vi "Switch_Manager_SoftFP.vi"(0 "reference in":refnum<class "Switch_Manager.lvclass">, 2 "Floating":bool, 5 "error in (no error)":errorcluster) -> (14 "reference out":refnum<class "Switch_Manager.lvclass">, 19 "error out":errorcluster)   [LabVIEW 2022 SP3, in "Switch_Manager.lvlib" / "Switch_Manager.lvclass"]
uses:
  Switch_Manager.lvclass
  <vilib>/picture/picture.llb/imagedata.ctl
  Components/ViPER.lvlibp/ViPER.lvclass
  C:/Projects/Medulla/ViPER/Examples/Flux_Capacitor_Tester/Components/ViPER.lvlibp/ViPER.lvclass
panel:
  in  "Disconnect":bool
  in  "Connect":bool
  in  "Tree":string(tree)
  in  "Disconnect_All":bool
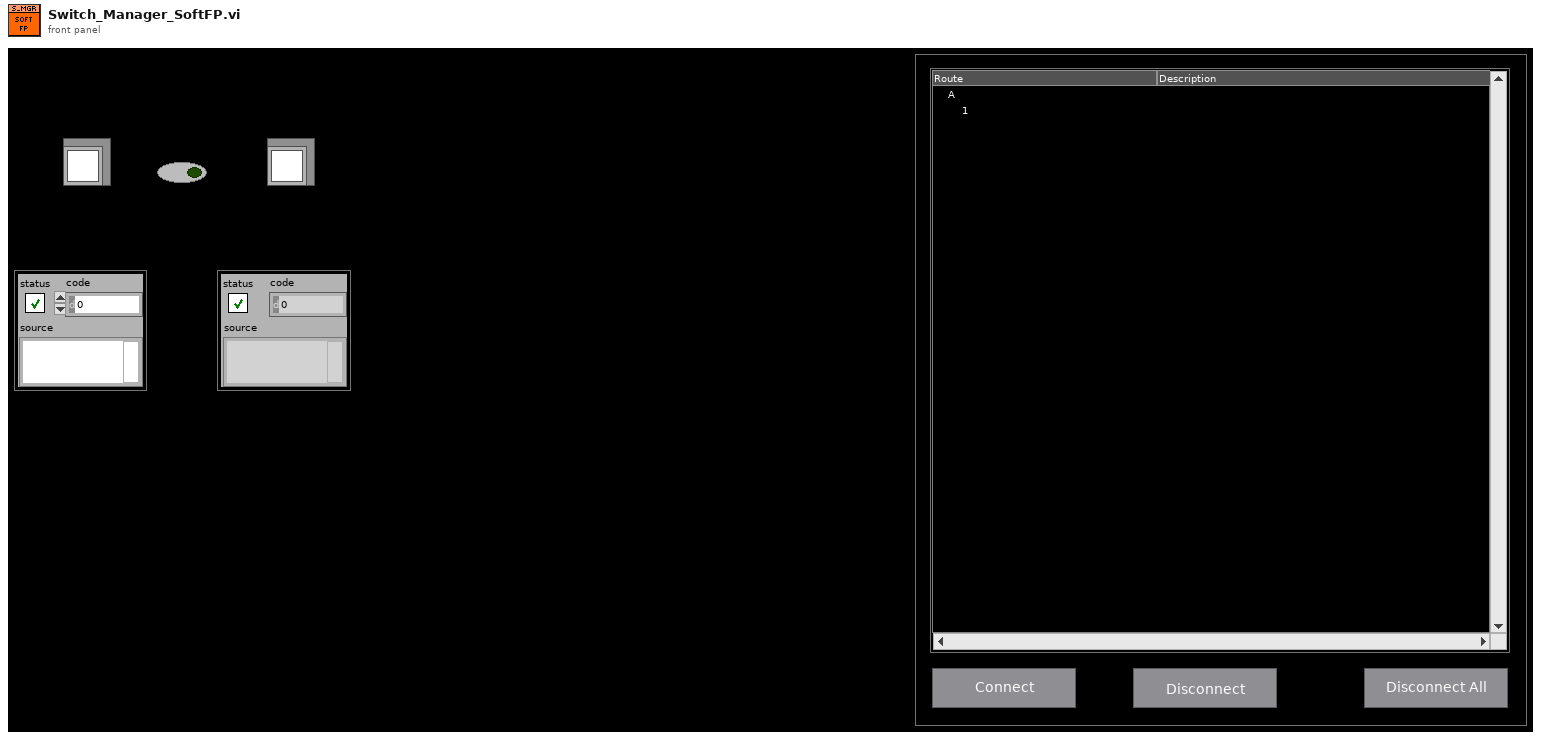
[diagram p1: front panel]
types:
  T1 = enum32{"Invalid", "Standard", "Closed", "Hidden", "Minimized", "Maximized"}
  T2 = typedef "Switch_Manager.lvlib/Switch_Manager.lvclass/ObjectAttributes.ctl" = cluster{"Config":T3, "State":bool[], "Switches":refnum<class "SwitchBase.lvclass">[], "SwitchName":string[], "SwitchMap":T4[], "UpdateEvent":refnum<user-event>, "ParentEvent":refnum<user-event>, "Tree":bool[]}
  T3 = typedef "Switch_Manager.lvlib/Switch_Manager.lvclass/Config.ctl" = cluster{"default":string}
  T4 = typedef "Switch_Manager.lvlib/Switch_Manager.lvclass/SwitchMap.ctl" = cluster{"Name":string, "Description":string, "Group":string, "IsGroup":bool, "Switches":string[]}
  T5 = typedef "imagedata.ctl" = cluster{"image type":i32, "image depth":i32, "image":u8[], "mask":u8[], "colors":u32[], "Rectangle":cluster{"left":i16, "top":i16, "right":i16, "bottom":i16}}
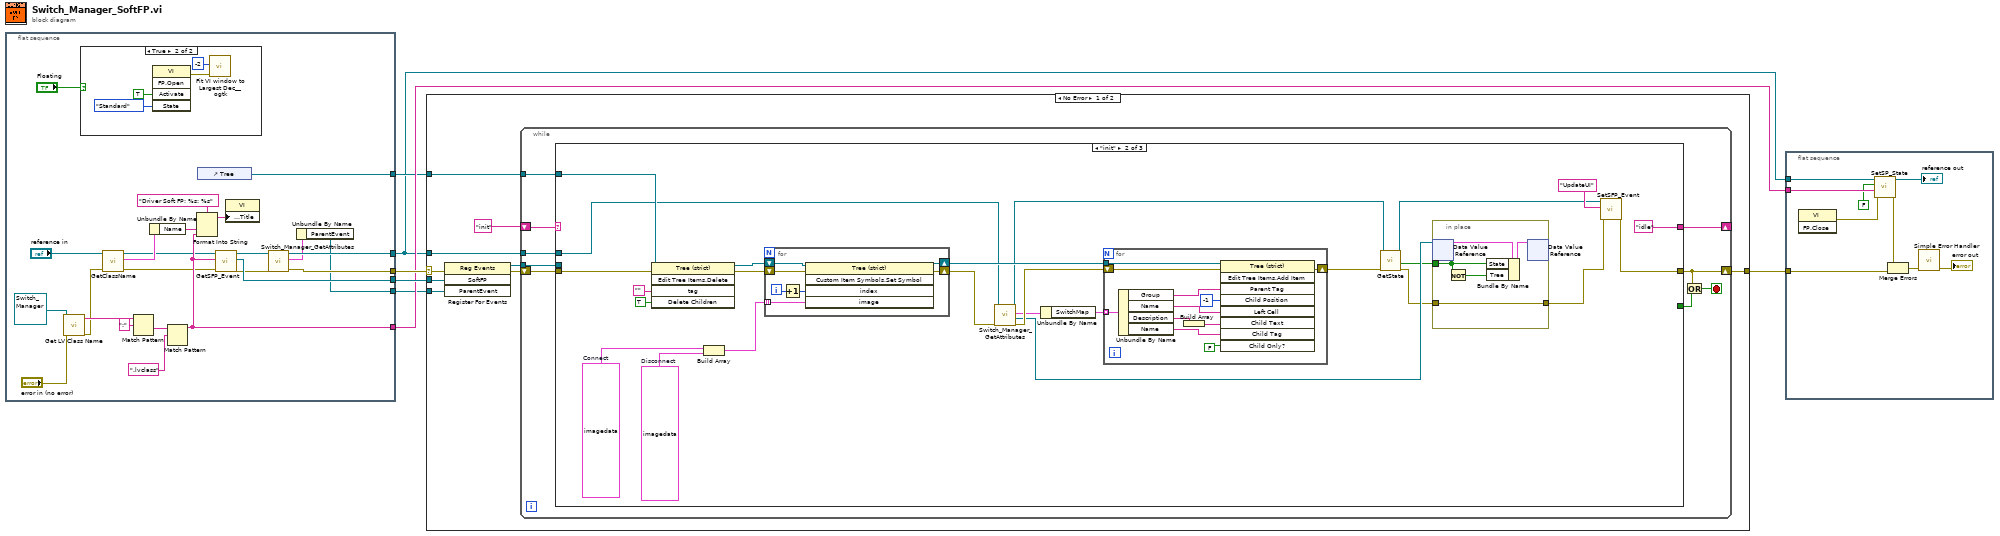
[diagram p0: block diagram]
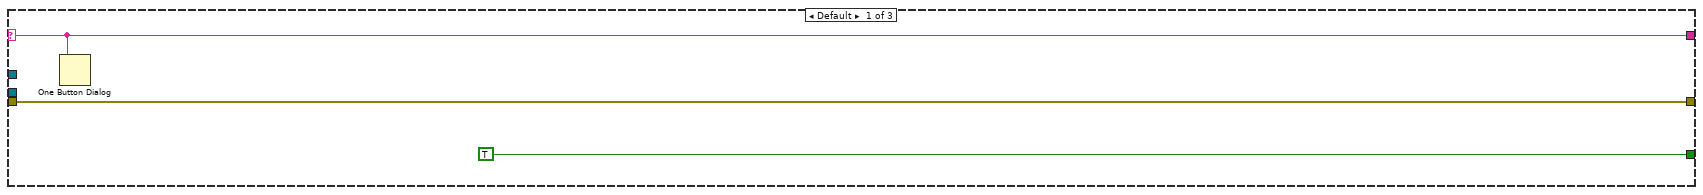
[diagram p3: hidden frame]
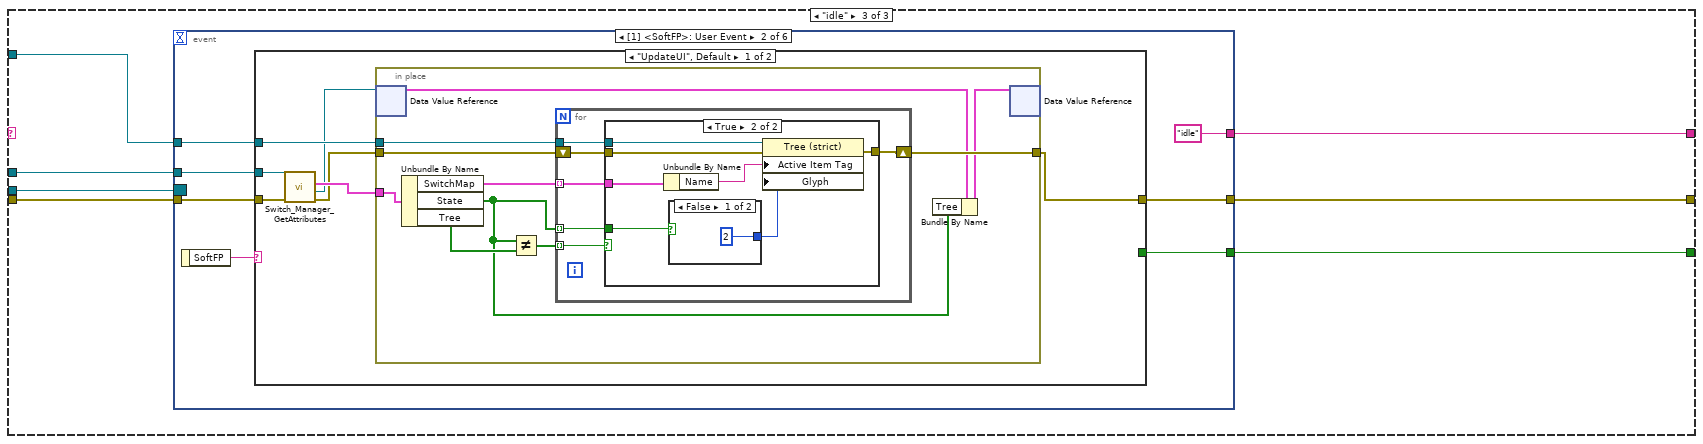
[diagram p4: hidden frame]
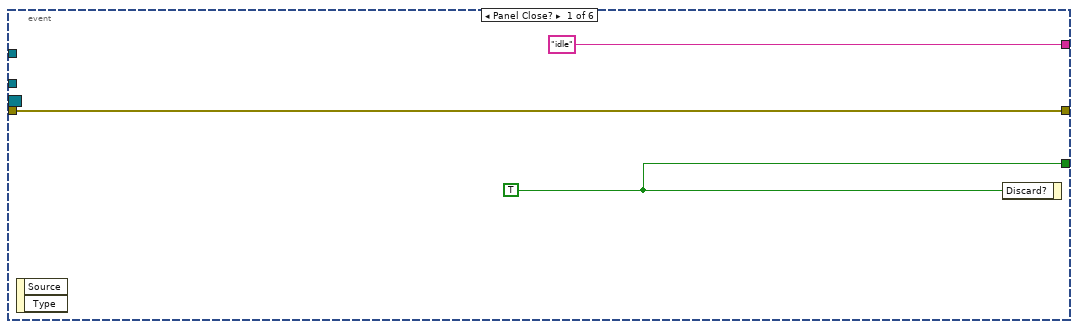
[diagram p5: hidden frame]
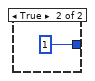
[diagram p7: hidden frame]
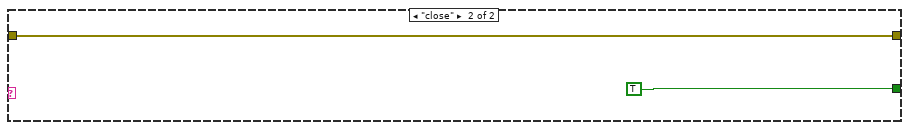
[diagram p8: hidden frame]
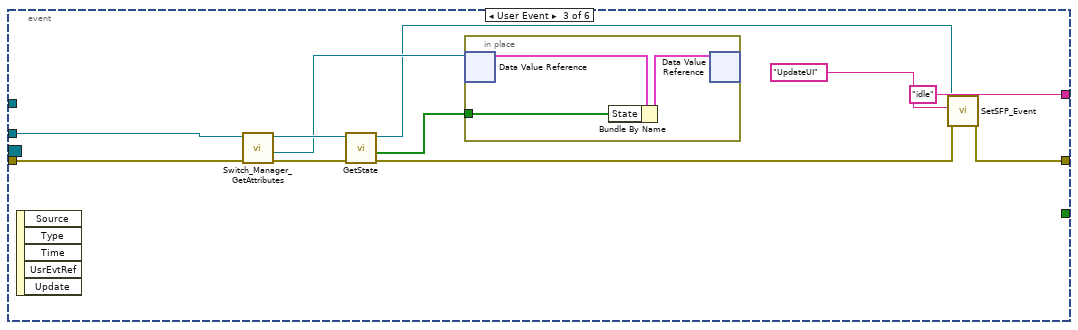
[diagram p9: hidden frame]
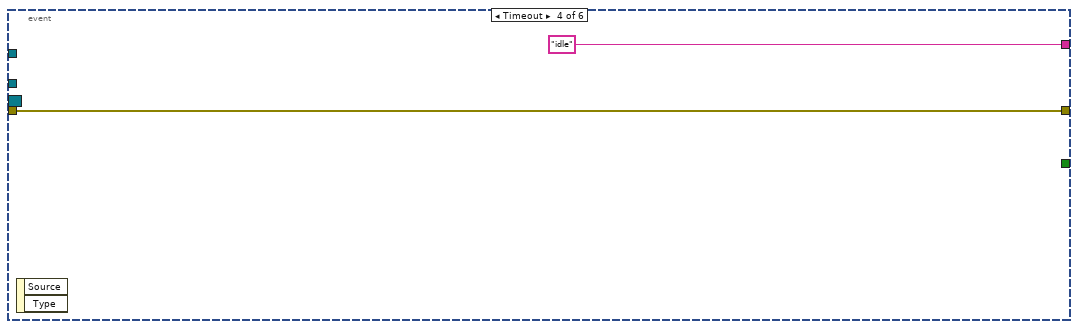
[diagram p10: hidden frame]
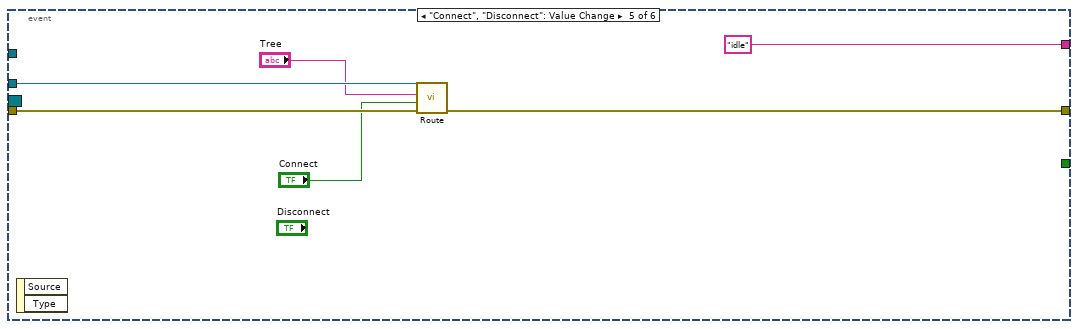
[diagram p11: hidden frame]
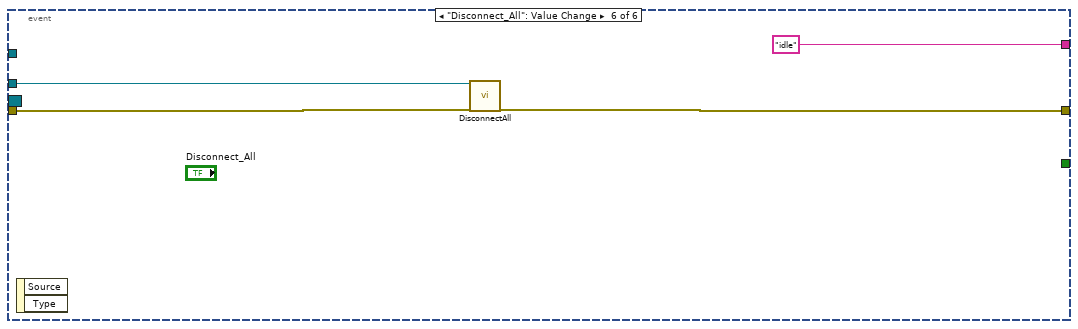
[diagram p12: hidden frame]
diagram:
  n1 = flat-sequence {
    tunnel: [w12] -> w7
    tunnel: [w10] -> w2
    tunnel: [w31] -> w5
    tunnel: [w21] -> w4
    tunnel: [w14] -> w3
    tunnel: [w8] -> w1
    frame #0 {
      n2 = call <vilib>:"Get LV Class Name.vi"("error in (no error)"="error in (no error)", "object"=refnum<class "Switch_Manager.lvclass"> refnum ("reference")) -> ("error out"=w20:errorcluster, "class name"=w26:string)  [unwired: 8 in]
      n3 = case shown="True" "Floating" {
        frame False {
        }
        frame True {
          n4 = invoke class="VI" method="FP.Open"("Activate"=TRUE ("Activate?"), "State"=T1."Standard") -> (error out=w32:errorcluster)  [unwired: 3 in, 4 out]
          n5 = call <userlib>:"Fit VI window to Largest Dec__ogtk.vi"("error in (no error)"=w32, "border spacing (2 px)"=-2) -> ()  [unwired: 4 in, 2 out]
        }
      }
      n6 = call "GetClassName.vi"("error in (no error)"=w20, "reference in"="reference in") -> ("error out"=w19:errorcluster, "Details"=w18:cluster{"Name":string, "Class":string}, "reference out"=w16:refnum<class "Switch_Manager.lvclass">)  [unwired: 7 in]
      n7 = Match Pattern(string=w26, regular expression=":") -> (after substring=w24:string)  [unwired: 1 in, 3 out]
      n8 = Unbundle By Name(w18) -> ("Name"=w28:string)
      n9 = Match Pattern(string=w24, regular expression=".lvclass") -> (before substring=w21:string)  [unwired: 1 in, 3 out]
      n10 = Format Into String(format string="Driver Soft FP: %s: %s", w28, w21) -> (resulting string=w30:string)  [unwired: 2 in, 1 out]
      n11 = control-ref of="Tree"() -> (w14:refnum<vi>)
      n12 = call-dynamic "GetSFP_Event.vi"("error in (no error)"=w19, "Ancestor"=w21, "reference in"=w16) -> ("error out"=w13:errorcluster, "SoftFP"=w31:refnum<user-event>, "reference out"=w11:refnum<class "Switch_Manager.lvclass">)  [unwired: 6 in]
      n13 = property class="VI"("Front Panel.Title"=w30) -> ()  [unwired: 2 in, 2 out]
      n14 = call "Switch_Manager_GetAttributes.vi"("error in (no error)"=w13, "reference in"=w11) -> ("error out"=w12:errorcluster, "Data"=w9:T2, "reference out"=w10:refnum<class "Switch_Manager.lvclass">)  [unwired: 6 in, 1 out]
      n15 = Unbundle By Name(w9) -> ("ParentEvent"=w8:refnum<user-event>)
    }
  }
  n16 = case shown="No Error" w7 {
    selector: w7 -> [w42 w183]
    tunnel: [w38 w183] -> w6
    tunnel: w2 -> [w39 _]
    tunnel: w5 -> [w44 _]
    tunnel: w3 -> [w37 _]
    tunnel: w1 -> [w36 _]
    frame No Error {
      n17 = register-events(error in=w42, w44, w36) -> (reference out=w43:refnum<event-registration>, error out=w41:errorcluster)  [unwired: 1 in]
      n18 = while {
        shift-right: [w50] -> w38
        shift-left: w41 -> [w53]
        tunnel: w43 -> [w52]
        tunnel: w39 -> [w51]
        shift-right: [w46] -> _
        shift-left: "init" -> [w47]
        tunnel: w37 -> [w45]
        stop <- w49 stop-if-true
        n19 = case shown="\"init\"" w47 {
          selector: w47 -> [w54 _ _]
          tunnel: w53 -> [w55 w71 w111]
          tunnel: w52 -> [_ _ w110]
          tunnel: w51 -> [_ w66 w109]
          tunnel: [w55 w80 w108] -> w50
          tunnel: [TRUE ("Discard?") _ w107] -> w48
          tunnel: [w54 "idle" w106] -> w46
          tunnel: w45 -> [_ w70 w105]
          frame Default {
            n20 = One Button Dialog(message=w54) -> ()  [unwired: 1 in, 1 out]
          }
          frame "init" {
            w72 = T5 {"image type"=0, "image depth"=32, "image"=[255, 0, 0, 0, 255, 0, 0, 0, 255, 0, 0, 0, 255, 0, 0, 0, 255, 0, 0, 0, 255, 0, 0, 0, 255, 0, 0, 0, 255, 0, 0, 0, 255, 0, 0, 0, 255, 0, 0, 0, 255, 0, 0, 0, 255, 0, 0, 0, 255, 0, 0, 0, 255, 0, 0, 0, 255, 0, 0, 0, 255, 0, 0, 0, 255, 0, 0, 0, 255, 0, 0, 0, 255, 0, 0, 0, 255, 0, 0, 0, 255, 136, 118, 121, 255, 113, 64, 72, 255, 122, 43, 52, 255, 138, 48, 56, 255, 136, 46, 54, 255, 120, 40, 49, 255, 113, 64, 72, 255, 0, 0, 0, 255, 0, 0, 0, 255, 0, 0, 0, 255, 0, 0, 0, 255, 0, 0, 0, 255, 0, 0, 0, 255, 0, 0, 0, 255, 0, 0, 0, 255, 119, 79, 86, 255, 137, 51, 59, 255, 189, 85, 89, 255, 201, 100, 103, 255, 201, 102, 105, 255, 198, 94, 97, 255, 194, 81, 84, 255, 180, 64, 69, 255, 130, 39, 48, 255, 121, 84, 90, 255, 0, 0, 0, 255, 0, 0, 0, 255, 0, 0, 0, 255, 0, 0, 0, 255, 0, 0, 0, 255, 119, 79, 86, 255, 161, 64, 71, 255, 202, 103, 106, 255, 209, 123, 126, 255, 211, 129, 132, 255, 208, 122, 125, 255, 203, 105, 109, 255, 196, 87, 90, 255, 192, 74, 78, 255, 189, 68, 72, 255, 150, 47, 54, 255, 121, 86, 92, 255, 0, 0, 0, 255, 0, 0, 0, 255, 0, 0, 0, 255, 136, 118, 121, 255, 137, 51, 59, 255, 202, 103, 106, 255, 211, 129, 132, 255, 214, 140, 142, 255, 212, 133, 136, 255, 205, 113, 116, 255, 196, 88, 92, 255, 190, 68, 72, 255, 188, 63, 67, 255, 189, 68, 72, 255, 190, 69, 73, 255, 129, 40, 49, 255, 0, 0, 0, 255, 0, 0, 0, 255, 0, 0, 0, 255, 113, 64, 72, 255, 188, 84, 88, 255, 207, 120, 122, 255, 213, 135, 138, 255, 211, 131, 133, 255, 205, 112, 115, 255, 195, 85, 88, 255, 186, 59, 63, 255, 181, 44, 48, 255, 181, 45, 49, 255, 187, 61, 65, 255, 191, 73, 77, 255, 177, 62, 67, 255, 114, 68, 76, 255, 0, 0, 0, 255, 0, 0, 0, 255, 122, 42, 51, 255, 199, 94, 98, 255, 207, 118, 121, 255, 207, 119, 122, 255, 201, 102, 105, 255, 193, 78, 82, 255, 185, 54, 58, 255, 178, 36, 41, 255, 176, 28, 33, 255, 178, 34, 39, 255, 185, 55, 59, 255, 192, 74, 78, 255, 191, 71, 75, 255, 117, 40, 50, 255, 0, 0, 0, 255, 0, 0, 0, 255, 136, 44, 53, 255, 197, 89, 92, 255, 201, 100, 103, 255, 197, 88, 92, 255, 189, 67, 71, 255, 182, 47, 52, 255, 177, 33, 38, 255, 174, 25, 30, 255, 174, 23, 28, 255, 177, 32, 37, 255, 185, 54, 58, 255, 192, 75, 79, 255, 192, 75, 79, 255, 128, 36, 46, 255, 0, 0, 0, 255, 0, 0, 0, 255, 134, 40, 49, 255, 192, 75, 79, 255, 192, 77, 80, 255, 187, 60, 64, 255, 180, 41, 46, 255, 176, 29, 34, 255, 174, 24, 28, 255, 174, 22, 27, 255, 174, 25, 30, 255, 179, 37, 42, 255, 187, 61, 65, 255, 194, 81, 85, 255, 193, 78, 81, 255, 128, 37, 46, 255, 0, 0, 0, 255, 0, 0, 0, 255, 119, 35, 45, 255, 188, 63, 67, 255, 187, 61, 66, 255, 182, 46, 51, 255, 177, 32, 36, 255, 174, 25, 30, 255, 174, 24, 29, 255, 175, 27, 32, 255, 178, 36, 40, 255, 184, 53, 57, 255, 192, 76, 80, 255, 197, 90, 93, 255, 193, 79, 82, 255, 117, 42, 52, 255, 0, 0, 0, 255, 0, 0, 0, 255, 112, 63, 71, 255, 176, 52, 57, 255, 186, 59, 63, 255, 183, 50, 54, 255, 180, 40, 44, 255, 178, 36, 40, 255, 179, 38, 42, 255, 182, 46, 50, 255, 187, 60, 64, 255, 193, 79, 83, 255, 199, 96, 99, 255, 199, 96, 99, 255, 178, 70, 75, 255, 115, 72, 79, 255, 0, 0, 0, 255, 0, 0, 0, 255, 0, 0, 0, 255, 129, 34, 44, 255, 186, 59, 63, 255, 187, 61, 66, 255, 186, 59, 63, 255, 186, 59, 63, 255, 188, 64, 68, 255, 192, 75, 78, 255, 197, 89, 92, 255, 201, 102, 105, 255, 202, 104, 107, 255, 197, 89, 93, 255, 127, 44, 53, 255, 0, 0, 0, 255, 0, 0, 0, 255, 0, 0, 0, 255, 0, 0, 0, 255, 121, 84, 90, 255, 149, 44, 51, 255, 188, 65, 69, 255, 191, 72, 76, 255, 193, 78, 82, 255, 195, 85, 89, 255, 198, 93, 97, 255, 201, 100, 104, 255, 201, 101, 104, 255, 197, 90, 93, 255, 148, 54, 62, 255, 124, 93, 98, 255, 0, 0, 0, 255, 0, 0, 0, 255, 0, 0, 0, 255, 0, 0, 0, 255, 0, 0, 0, 255, 121, 85, 91, 255, 128, 38, 47, 255, 177, 61, 66, 255, 191, 73, 77, 255, 193, 79, 83, 255, 195, 83, 86, 255, 194, 82, 86, 255, 178, 71, 76, 255, 127, 44, 53, 255, 124, 93, 98, 255, 0, 0, 0, 255, 0, 0, 0, 255, 0, 0, 0, 255, 0, 0, 0, 255, 0, 0, 0, 255, 0, 0, 0, 255, 0, 0, 0, 255, 0, 0, 0, 255, 114, 68, 76, 255, 117, 40, 49, 255, 129, 37, 46, 255, 128, 37, 46, 255, 117, 42, 52, 255, 115, 72, 79, 255, 0, 0, 0, 255, 0, 0, 0, 255, 0, 0, 0, 255, 0, 0, 0, 255, 0, 0, 0, 255, 0, 0, 0, 255, 0, 0, 0, 255, 0, 0, 0, 255, 0, 0, 0, 255, 0, 0, 0, 255, 0, 0, 0, 255, 0, 0, 0, 255, 0, 0, 0, 255, 0, 0, 0, 255, 0, 0, 0, 255, 0, 0, 0, 255, 0, 0, 0, 255, 0, 0, 0, 255, 0, 0, 0, 255, 0, 0, 0, 255, 0, 0, 0], "mask"=[255, 255, 255, 255, 255, 255, 255, 255, 255, 255, 255, 255, 255, 255, 255, 255, 255, 255, 255, 255, 255, 255, 255, 255, 255, 255, 255, 255, 255, 255, 255, 255], "colors"=[], "Rectangle"={"left"=0, "top"=0, "right"=16, "bottom"=16}}  # Disconnect
            w73 = T5 {"image type"=0, "image depth"=32, "image"=array[1024 elements], "mask"=[255, 255, 255, 255, 255, 255, 255, 255, 255, 255, 255, 255, 255, 255, 255, 255, 255, 255, 255, 255, 255, 255, 255, 255, 255, 255, 255, 255, 255, 255, 255, 255], "colors"=[], "Rectangle"={"left"=0, "top"=0, "right"=16, "bottom"=16}}  # Connect
            n21 = invoke class="Tree (strict)" method="Edit Tree Items.Delete"(reference=w70, error in=w71, "tag"="", "Delete Children"=TRUE ("Delete Children?")) -> (reference out=w74:refnum<vi>, error out=w75:errorcluster)  [unwired: 1 in, 3 out]
            n22 = Build Array(w73, w72) -> (w78:T5[])
            n23 = for {
              tunnel: w78 -> [w101] mode=indexing
              shift-right: [w100] -> w68
              shift-left: w75 -> [w103]
              shift-right: [w98] -> w69
              shift-left: w74 -> [w99]
              i -> [w104]
              n24 = Increment(x=w104) -> (x+1=w102:i32)
              n25 = invoke class="Tree (strict)" method="Custom Item Symbols.Set Symbol"(reference=w99, error in=w103, "index"=w102, "image"=w101) -> (reference out=w98:refnum<vi>, error out=w100:errorcluster)  [unwired: 1 in, 3 out]
            }
            n26 = call "Switch_Manager_GetAttributes.vi"("error in (no error)"=w68, "reference in"=w66) -> ("error out"=w67:errorcluster, "DataRef"=w60:refnum<data-value>, "Data"=w65:T2, "reference out"=w62:refnum<class "Switch_Manager.lvclass">)  [unwired: 6 in]
            n27 = Unbundle By Name(w65) -> ("SwitchMap"=w64:T4[])
            n28 = for {
              tunnel: w64 -> [w97] mode=indexing
              tunnel: w69 -> [w90]
              shift-right: [w88] -> w63
              shift-left: w67 -> [w89]
              n29 = Unbundle By Name(w97) -> ("Group"=w96:string, "Name"=w92:string, "Description"=w94:string, "Name"=w87:string)
              n30 = Build Array(w94) -> (w93:string[])
              n31 = invoke class="Tree (strict)" method="Edit Tree Items.Add Item"(reference=w90, error in=w89, "Parent Tag"=w96, "Child Position"=-1, "Left Cell"=w92, "Child Text"=w93, "Child Tag"=w87, "Child Only?"=FALSE) -> (error out=w88:errorcluster)  [unwired: 1 in, 8 out]
            }
            n32 = call-dynamic "GetState.vi"("error in (no error)"=w63, "reference in"=w62) -> ("error out"=w58:errorcluster, "States"=w59:bool[], "reference in"=w61:refnum<class "Switch_Manager.lvclass">)  [unwired: 6 in, 1 out]
            n33 = in-place {
              in-place-border: w58 -> [w84]
              in-place-border: w59 -> [w83]
              in-place-border: [w84] -> w57
              n34 = in-place-dvr #1(w60) -> (w86:T2)  [unwired: 1 out]
              n35 = Not(x=w83) -> (.not. x?=w82:bool[])
              n36 = Bundle By Name(cluster=w86, "State"=w83, "Tree"=w82) -> (w85:T2)
              n37 = in-place-dvr #1(w85) -> ()  [unwired: 2 out]
            }
            n38 = call-dynamic "SetSFP_Event.vi"("error in (no error)"=w57, "msg"="UpdateUI", "reference in"=w61) -> ("error out"=w80:errorcluster)  [unwired: 7 in, 1 out]
          }
          frame "idle" {
            n39 = event shown="[1] <SoftFP>: User Event" {
              selector: w110 -> [_ _ _ _ _ _]
              dyn-events: _ -> [_ _ _ _ _ _]
              timeout: _ -> [_ _ _ _ _ _]
              tunnel: w111 -> [w114 w121 w166 w172 w177 w181]
              tunnel: [w114 w119 w157 w172 w176 w179] -> w108
              tunnel: [w113 w118 _ _ _ _] -> w107
              tunnel: w109 -> [_ w116 w164 _ w175 w180]
              tunnel: ["idle" "idle" "idle" "idle" "idle" "idle"] -> w106
              tunnel: w105 -> [_ w115 _ _ _ _]
              event Panel Close? {
                w113 = TRUE ("Discard?")
                n40 = event-data() -> ()  [unwired: 1 in, 2 out]
                n41 = event-data("Discard?"=w113) -> ()  [unwired: 1 in, 1 out]
              }
              event User Event {
                n42 = event-data() -> ("SoftFP"=w120:string)  [unwired: 1 in]
                n43 = case shown="\"UpdateUI\", Default" w120 {
                  tunnel: w121 -> [w128 w156]
                  tunnel: [w124 w156] -> w119
                  tunnel: [_ TRUE ("Discard?")] -> w118
                  tunnel: w116 -> [w127 _]
                  tunnel: w115 -> [w123 _]
                  frame "UpdateUI", Default {
                    n44 = call "Switch_Manager_GetAttributes.vi"("error in (no error)"=w128, "reference in"=w127) -> ("error out"=w125:errorcluster, "DataRef"=w122:refnum<data-value>, "Data"=w126:T2)  [unwired: 6 in, 1 out]
                    n45 = in-place {
                      in-place-border: w126 -> [w138]
                      in-place-border: w125 -> [w136]
                      in-place-border: [w135] -> w124
                      in-place-border: w123 -> [w134]
                      n46 = in-place-dvr #2(w122) -> (w131:T2)  [unwired: 1 out]
                      n47 = Unbundle By Name(w138) -> ("SwitchMap"=w137:T4[], "State"=w129:bool[], "Tree"=w133:bool[])
                      n48 = Not Equal?(x=w129, y=w133) -> (x != y?=w132:bool[])
                      n49 = for {
                        tunnel: w137 -> [w144] mode=indexing
                        tunnel: w129 -> [w143] mode=indexing
                        shift-right: [w141] -> w135
                        shift-left: w136 -> [w142]
                        tunnel: w134 -> [w140]
                        tunnel: w132 -> [w139] mode=indexing
                        n50 = case shown="True" w139 {
                          tunnel: w144 -> [_ w152]
                          tunnel: w143 -> [_ w146]
                          tunnel: w142 -> [w145 w149]
                          tunnel: [w145 w148] -> w141
                          tunnel: w140 -> [_ w147]
                          frame False {
                          }
                          frame True {
                            n51 = Unbundle By Name(w152) -> ("Name"=w151:string)
                            n52 = case shown="False" w146 {
                              tunnel: [2 1] -> w150
                              frame False {
                              }
                              frame True {
                              }
                            }
                            n53 = property class="Tree (strict)"(reference=w147, error in=w149, "Active Item Tag"=w151, "Glyph"=w150) -> (error out=w148:errorcluster)  [unwired: 1 out]
                          }
                        }
                      }
                      n54 = Bundle By Name(cluster=w131, "Tree"=w129) -> (w130:T2)
                      n55 = in-place-dvr #2(w130) -> ()  [unwired: 2 out]
                    }
                  }
                  frame "close" {
                  }
                }
              }
              event User Event {
                n56 = event-data() -> ()  [unwired: 1 in, 5 out]
                n57 = call "Switch_Manager_GetAttributes.vi"("error in (no error)"=w166, "reference in"=w164) -> ("error out"=w167:errorcluster, "DataRef"=w163:refnum<data-value>, "reference out"=w165:refnum<class "Switch_Manager.lvclass">)  [unwired: 6 in, 1 out]
                n58 = call-dynamic "GetState.vi"("error in (no error)"=w167, "reference in"=w165) -> ("error out"=w158:errorcluster, "States"=w162:bool[], "reference in"=w159:refnum<class "Switch_Manager.lvclass">)  [unwired: 6 in, 1 out]
                n59 = in-place {
                  in-place-border: w162 -> [w168]
                  n60 = in-place-dvr #3(w163) -> (w169:T2)  [unwired: 1 out]
                  n61 = Bundle By Name(cluster=w169, "State"=w168) -> (w170:T2)
                  n62 = in-place-dvr #3(w170) -> ()  [unwired: 2 out]
                }
                n63 = call-dynamic "SetSFP_Event.vi"("error in (no error)"=w158, "msg"="UpdateUI", "reference in"=w159) -> ("error out"=w157:errorcluster)  [unwired: 7 in, 1 out]
              }
              event Timeout {
                n64 = event-data() -> ()  [unwired: 1 in, 2 out]
              }
              event "Connect", "Disconnect": Value Change {
                n65 = event-data() -> ()  [unwired: 1 in, 2 out]
                n66 = call-dynamic "Route.vi"("error in (no error)"=w177, "Connect"="Connect", "Route"="Tree", "reference in"=w175) -> ("error out"=w176:errorcluster)  [unwired: 6 in, 1 out]
              }
              event "Disconnect_All": Value Change {
                n67 = event-data() -> ()  [unwired: 1 in, 2 out]
                n68 = call-dynamic "DisconnectAll.vi"("reference in"=w180, "error in (no error)"=w181) -> ("error out"=w179:errorcluster)  [unwired: 16 in, 1 out]
              }
            }
          }
        }
        n69 = Or(x=w50, y=w48) -> (x .or. y?=w49:bool)
      }
    }
    frame Error {
    }
  }
  n70 = flat-sequence {
    tunnel: w6 -> [w190]
    tunnel: w4 -> [w187]
    tunnel: w2 -> [w184]
    frame #0 {
      n71 = invoke class="VI" method="FP.Close"() -> (error out=w189:errorcluster)  [unwired: 3 in, 2 out]
      n72 = call "SetSP_State.vi"("error in (no error)"=w189, "Ancestor"=w187, "SP Open"=FALSE, "reference in"=w184) -> ("error out"=w188:errorcluster, "reference out"=→"reference out":refnum<class "Switch_Manager.lvclass">)  [unwired: 6 in]
      n73 = Merge Errors(w188, w190) -> (w192:errorcluster)
      n74 = call <vilib>:"Simple Error Handler.vi"("error in (no error)"=w192) -> ("error out"=→"error out":errorcluster)  [unwired: 4 in, 4 out]
    }
  }
